vi "readCommandManipulateM1M3.vi"(8 "error in (no error)":errorcluster, 10 "Parser":refnum<class "U8ArrayParserAutoIndexing.lvclass">, 11 "M1M3SAL in":refnum<class "M1M3SAL.lvclass">) -> (0 "error out":errorcluster, 2 "CommandManipulateM1M3":variant, 3 "M1M3SAL out":refnum<class "M1M3SAL.lvclass">)   [LabVIEW 2016, in "M1M3SupportCommunicator.lvlib" / "M1M3SAL.lvclass"]
uses:
  M1M3SAL.lvclass
  Common_RT_Utilities/U8ArrayParserAutoIndexing/U8ArrayParserAutoIndexing.lvclass
  DataTypes/Topics/CommandManipulateM1M3.ctl
  DataTypes/Topics/Parts/CommandId.ctl
  DataTypes/Topics/M1M3SupportTopics.lvlib
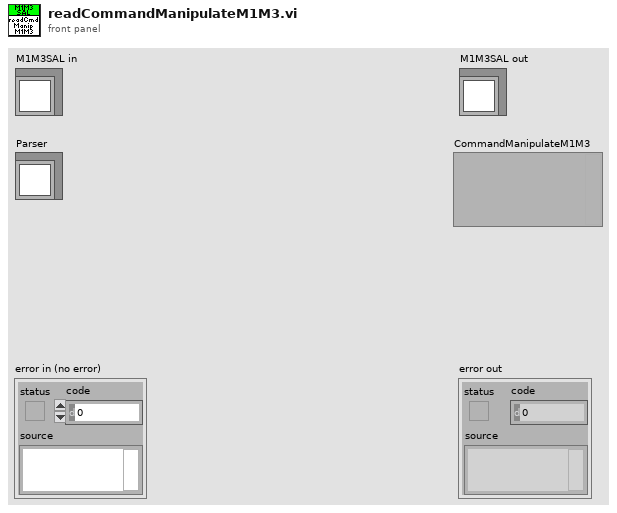
[diagram p1: front panel]
types:
  T1 = typedef "M1M3SupportTopics.lvlib/CommandManipulateM1M3.ctl" = cluster{"CommandId":T2, "XTranslation":dbl, "YTranslation":dbl, "ZTranslation":dbl, "XRotation":dbl, "YRotation":dbl, "ZRotation":dbl}
  T2 = typedef "M1M3SupportTopics.lvlib/CommandId.ctl" = i32
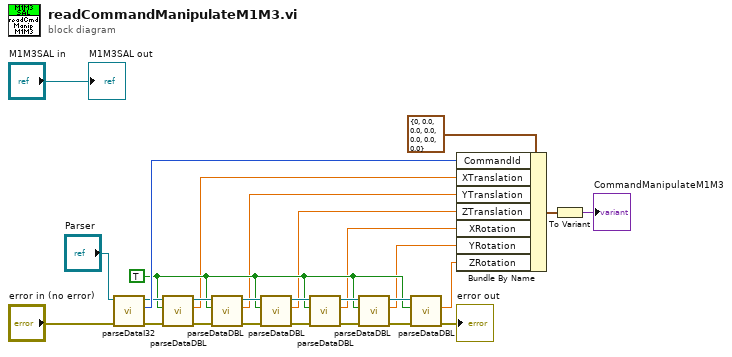
[diagram p0: block diagram]
diagram:
  w8 = TRUE ("OverrideSwapBytes")
  n1 = call "parseDataI32.vi"("error in (no error)"="error in (no error)", "U8ArrayParserAutoIndexing in"="Parser") -> ("error out"=w9:errorcluster, "Data"=w23:i32, "U8ArrayParserAutoIndexing out"=w18:refnum<class "U8ArrayParserAutoIndexing.lvclass">)  [unwired: 7 in]
  n2 = call "parseDataDBL.vi"("error in (no error)"=w9, "OverrideSwapBytes"=w8, "U8ArrayParserAutoIndexing in"=w18) -> ("error out"=w10:errorcluster, "Data"=w1:dbl, "U8ArrayParserAutoIndexing out"=w17:refnum<class "U8ArrayParserAutoIndexing.lvclass">)  [unwired: 6 in]
  n3 = call "parseDataDBL.vi"("error in (no error)"=w10, "OverrideSwapBytes"=w8, "U8ArrayParserAutoIndexing in"=w17) -> ("error out"=w11:errorcluster, "Data"=w2:dbl, "U8ArrayParserAutoIndexing out"=w16:refnum<class "U8ArrayParserAutoIndexing.lvclass">)  [unwired: 6 in]
  n4 = call "parseDataDBL.vi"("error in (no error)"=w11, "OverrideSwapBytes"=w8, "U8ArrayParserAutoIndexing in"=w16) -> ("error out"=w12:errorcluster, "Data"=w3:dbl, "U8ArrayParserAutoIndexing out"=w15:refnum<class "U8ArrayParserAutoIndexing.lvclass">)  [unwired: 6 in]
  n5 = call "parseDataDBL.vi"("error in (no error)"=w12, "OverrideSwapBytes"=w8, "U8ArrayParserAutoIndexing in"=w15) -> ("error out"=w13:errorcluster, "Data"=w4:dbl, "U8ArrayParserAutoIndexing out"=w14:refnum<class "U8ArrayParserAutoIndexing.lvclass">)  [unwired: 6 in]
  n6 = call "parseDataDBL.vi"("error in (no error)"=w13, "OverrideSwapBytes"=w8, "U8ArrayParserAutoIndexing in"=w14) -> ("error out"=w20:errorcluster, "Data"=w5:dbl, "U8ArrayParserAutoIndexing out"=w19:refnum<class "U8ArrayParserAutoIndexing.lvclass">)  [unwired: 6 in]
  n7 = call "parseDataDBL.vi"("error in (no error)"=w20, "OverrideSwapBytes"=w8, "U8ArrayParserAutoIndexing in"=w19) -> ("error out"=→"error out":errorcluster, "Data"=w6:dbl)  [unwired: 6 in, 1 out]
  n8 = Bundle By Name(cluster=T1 {"CommandId"=0, "XTranslation"=0.0, "YTranslation"=0.0, "ZTranslation"=0.0, "XRotation"=0.0, "YRotation"=0.0, "ZRotation"=0.0} ("CommandManipulateM1M3"), "CommandId"=w23, "XTranslation"=w1, "YTranslation"=w2, "ZTranslation"=w3, "XRotation"=w4, "YRotation"=w5, "ZRotation"=w6) -> (w26:T1)
  n9 = To Variant(anything=w26) -> (Variant=→"CommandManipulateM1M3":variant)
  "M1M3SAL out" <- "M1M3SAL in"
